vi "Lift_State_Machine.vi"() -> ()   [LabVIEW 2016]
doc: "The state machine for the Lift System.\nDrives the lift forward, then upward, then down, then back to its origin."
uses:
  <vilib>/myRIO/Instrument Drivers/Onboard IO/DIO/typedefs/DIO Reference.ctl
  <vilib>/myRIO/Common/Instrument Driver Framework/Utilities/typedefs/myRIO Generic Hardware Reference.ctl
  <vilib>/myRIO/Common/Instrument Driver Framework/Utilities/typedefs/Hardware Version Enum.ctl
  <vilib>/myRIO/Common/Instrument Driver Framework/Utilities/typedefs/myRIO v1.0 Reference.ctl
  <vilib>/myRIO/Common/Instrument Driver Framework/Utilities/typedefs/Generic FPGA Reference.ctl
  <vilib>/myRIO/Common/Instrument Driver Framework/myRIO v1.0/DIO/typedefs/DIO Channels List.ctl
  <vilib>/myRIO/Common/Instrument Driver Framework/myRIO v1.0/DIO/typedefs/DIO Channels Enum.ctl
  <vilib>/userdefined/High Color/nirio_resource_hc.ctl
  <vilib>/myRIO/Instrument Drivers/Onboard IO/AI/typedefs/AI Reference.ctl
  <vilib>/myRIO/Common/Instrument Driver Framework/myRIO v1.0/AI/typedefs/AI Channels List.ctl
  <vilib>/myRIO/Common/Instrument Driver Framework/myRIO v1.0/AI/typedefs/AI Channels Enum.ctl
  <vilib>/myRIO/Common/Instrument Driver Framework/Utilities/typedefs/Analog Scaling Constants List.ctl
  <vilib>/myRIO/Common/Instrument Driver Framework/Utilities/typedefs/Analog Scaling Constants.ctl
  <vilib>/myRIO/Common/Instrument Driver Framework/Utilities/vis/Is FPGA Ref Available.vi
  <vilib>/myRIO/Common/Instrument Driver Framework/roboRIO v1.0/DIO/vis/roboRIO v1.0 Open DIO.vi
  <vilib>/myRIO/Instrument Drivers/Onboard IO/DIO/vis/Write.vi
  <vilib>/myRIO/Instrument Drivers/Onboard IO/DIO/vis/Read.vi
  <vilib>/myRIO/Common/Instrument Driver Framework/roboRIO v1.0/AI/vis/roboRIO v1.0 Open AI.vi
  <vilib>/myRIO/Instrument Drivers/Onboard IO/AI/vis/Read.vi
  <vilib>/myRIO/Common/Instrument Driver Framework/Utilities/vis/Validate Channels.vi
  <vilib>/myRIO/Common/Instrument Driver Framework/roboRIO v1.0/DIO/vis/roboRIO v1.0 Reserve DIO.vi
  <vilib>/myRIO/Common/Instrument Driver Framework/roboRIO v1.0/AI/vis/roboRIO v1.0 Reserve AI.vi
  <vilib>/myRIO/Common/Instrument Driver Framework/roboRIO v1.0/DIO/vis/roboRIO v1.0 Build MUX Configuration DIO.vi
  <vilib>/myRIO/Common/Instrument Driver Framework/roboRIO v1.0/Resource Manager/vis/roboRIO v1.0 Reserve Channel List.vi
  <vilib>/myRIO/Common/Instrument Driver Framework/roboRIO v1.0/AI/vis/roboRIO v1.0 Build MUX Configuration AI.vi
  <vilib>/myRIO/Common/Instrument Driver Framework/roboRIO v1.0/Resource Manager/vis/roboRIO v1.0 Create Configuration List.vi
  <vilib>/myRIO/Common/Instrument Driver Framework/roboRIO v1.0/Resource Manager/vis/roboRIO v1.0 Reserve Channel.vi
  <vilib>/myRIO/Common/Instrument Driver Framework/roboRIO v1.0/Resource Manager/vis/roboRIO v1.0 Unreserve Channel.vi
  <vilib>/myRIO/Common/Instrument Driver Framework/roboRIO v1.0/Resource Manager/vis/roboRIO v1.0 Build Mutex Name.vi
  <vilib>/Utility/VariantDataType/GetNumericInfo.vi
  <vilib>/Utility/error.llb/Error Cluster From Error Code.vi
  <vilib>/myRIO/Common/Instrument Driver Framework/roboRIO v1.0/roboRIO v1.0 Open.vi
  <vilib>/myRIO/Common/Instrument Driver Framework/Utilities/vis/IO Manager.vi
  <vilib>/myRIO/Common/Instrument Driver Framework/Utilities/vis/Configuration Manager.vi
  <vilib>/myRIO/Common/Instrument Driver Framework/roboRIO v1.0/Resource Manager/vis/roboRIO v1.0 Configure IO.vi
  <vilib>/myRIO/Common/Instrument Driver Framework/myRIO v1.0/myRIO v1.0 Close.vi
  <vilib>/myRIO/Common/Instrument Driver Framework/roboRIO v1.0/DIO/vis/roboRIO v1.0 Write DIO.vi
  <vilib>/myRIO/Common/Instrument Driver Framework/roboRIO v1.0/DIO/vis/roboRIO v1.0 Read DIO.vi
  <vilib>/myRIO/Common/Instrument Driver Framework/roboRIO v1.0/AI/vis/roboRIO v1.0 Get Scaling Constants AI.vi
  <vilib>/myRIO/Common/Instrument Driver Framework/roboRIO v1.0/AI/vis/roboRIO v1.0 Read AI.vi
  <vilib>/myRIO/Express VI/Onboard IO/DO/DO Express VI.xnode
  <vilib>/myRIO/Instrument Drivers/Onboard IO/DIO/vis/myRIO DIO Open.xnode
  <vilib>/myRIO/Express VI/Onboard Devices/Button/Button Express VI.xnode
  <vilib>/myRIO/Express VI/Onboard Devices/LED/LED Express VI.xnode
  <vilib>/myRIO/Express VI/Onboard IO/AI/AI Express VI.xnode
  <vilib>/myRIO/Instrument Drivers/Onboard IO/AI/vis/myRIO AI Open.xnode
  <vilib>/myRIO/Instrument Drivers/Onboard IO/DIO/DIO.lvlib
  <vilib>/myRIO/Instrument Drivers/Onboard IO/AI/AI.lvlib
panel:
  in  "State change delay":dbl=1.0 caption="Delay Time (s)"
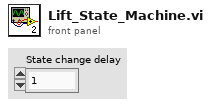
[diagram p1: front panel]
types:
  T1 = typedef "DIO.lvlib/DIO Reference.ctl" = cluster{"myRIO Reference":T2, "DIO Channels List":T6}
  T2 = typedef "myRIO Generic Hardware Reference.ctl" = cluster{"myRIO Model":T3, "myRIO Hardware Reference":T4}
  T3 = typedef "Hardware Version Enum.ctl" = enum16{"Unknown", "myRIO-1900", "myRIO-1950", "roboRIO", "NI ELVIS RIO CM"}
  T4 = typedef "myRIO v1.0 Reference.ctl" = cluster{"Generic FPGA Reference":T5, "Allow multiple opens":bool}
  T5 = typedef "Generic FPGA Reference.ctl" = refnum<k20>
  T6 = typedef "DIO Channels List.ctl" = T7[]
  T7 = typedef "DIO Channels Enum.ctl" = enum16{"Not Connected", "C/DIO0", "C/DIO1", "C/DIO2", "C/DIO3", "C/DIO4", "C/DIO5", "C/DIO6", "C/DIO7", "A/DIO0", "A/DIO1", "A/DIO2", "A/DIO3", "A/DIO4", "A/DIO5", "A/DIO6", "A/DIO7", "A/DIO8", "A/DIO9", "A/DIO10", "A/DIO11", "A/DIO12", "A/DIO13", "A/DIO14", "A/DIO15", "B/DIO0", "B/DIO1", "B/DIO2", "B/DIO3", "B/DIO4", "B/DIO5", "B/DIO6", "B/DIO7", "B/DIO8", "B/DIO9", "B/DIO10", "B/DIO11", "B/DIO12", "B/DIO13", "B/DIO14", "B/DIO15", "LED0", "LED1", "LED2", "LED3", "Button0", "DIO/DIO0", "DIO/DIO1", "DIO/DIO2", "DIO/DIO3", "DIO/DIO4", "DIO/DIO5", "DIO/DIO6", "DIO/DIO7", "DIO/DIO8", "DIO/DIO9", "SPI/CS0", "SPI/CS1", "SPI/CS2", "SPI/CS3", "LED RADIO (Green)", "LED RADIO (Red)", "LED COMM (Green)", "LED COMM (Red)", "LED MODE (Green)", "LED MODE (Red)"}
  T8 = typedef "nirio_resource_hc.ctl" = tag
  T9 = typedef "AI.lvlib/AI Reference.ctl" = cluster{"myRIO Reference":T2, "AI Channels List":T10, "AI Scaling Constants List":T12}
  T10 = typedef "AI Channels List.ctl" = T11[]
  T11 = typedef "AI Channels Enum.ctl" = enum16{"Not Connected", "AudioIn/Left", "AudioIn/Right", "C/AI0", "C/AI1", "A/AI0", "A/AI1", "A/AI2", "A/AI3", "B/AI0", "B/AI1", "B/AI2", "B/AI3", "AI/AI0", "AI/AI1", "AI/AI2", "AI/AI3"}
  T12 = typedef "Analog Scaling Constants List.ctl" = T13[]
  T13 = typedef "Analog Scaling Constants.ctl" = cluster{"LSB Weight (Volts)":dbl, "Offset (Volts)":dbl, "Signed?":bool}
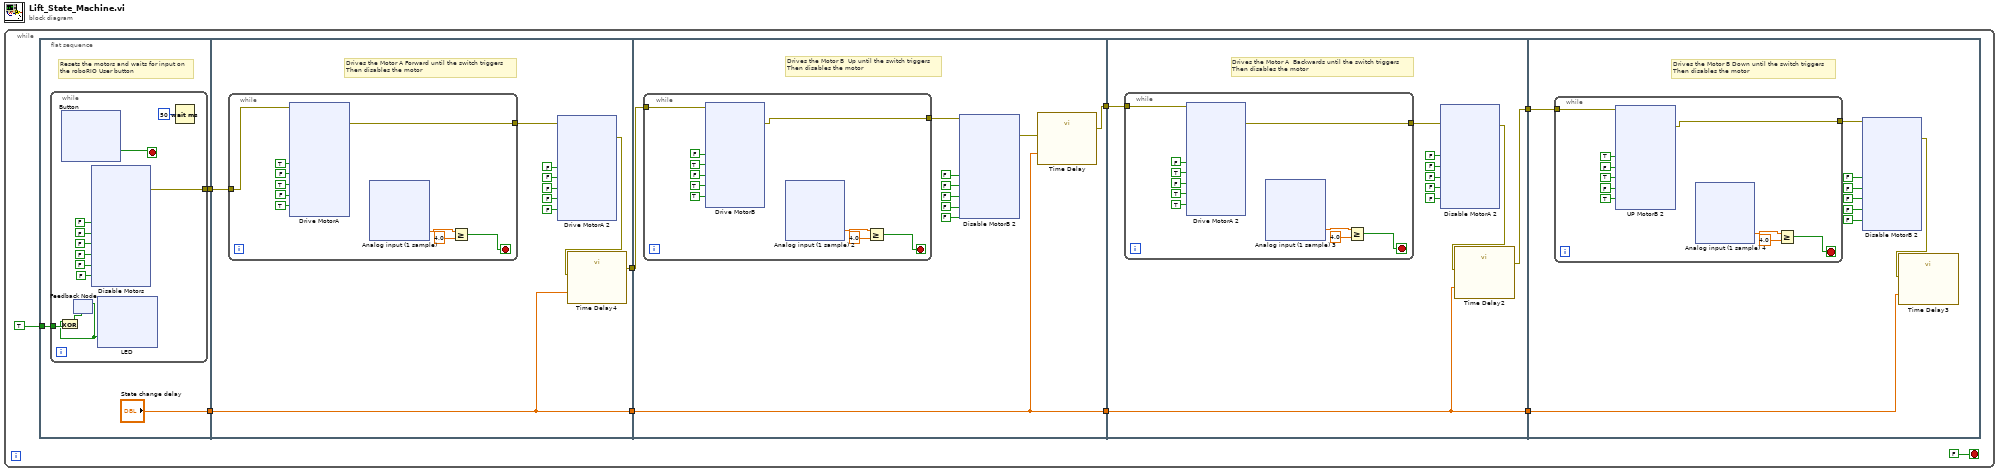
[diagram p0: block diagram]
diagram:
  n1 = while {
    stop <- FALSE stop-if-true
    n2 = flat-sequence {
      tunnel: ["State change delay"] -> w10
      tunnel: [w12] -> w9
      tunnel: TRUE -> [w11]
      tunnel: w10 -> [w138]
      tunnel: [w138] -> w8
      tunnel: [w137] -> w7
      tunnel: w9 -> [w136]
      tunnel: w8 -> [w273]
      tunnel: [w273] -> w6
      tunnel: w7 -> [w272]
      tunnel: [w271] -> w5
      tunnel: w6 -> [w408]
      tunnel: [w408] -> w4
      tunnel: w5 -> [w407]
      tunnel: [w406] -> w3
      tunnel: w4 -> [w542]
      tunnel: w3 -> [w541]
      frame #0 {
        # "Resets the motors and waits for input on\nthe roboRIO User button"
        n3 = while {
          tunnel: [w19] -> w12
          tunnel: w11 -> [w17]
          stop <- w18 stop-if-true
          n4 = xnode "Button"() -> ("Value"=w18:bool)  [unwired: 1 in, 1 out]
          n5 = feedback #1() -> (w15:bool)  [unwired: 1 in]
          n6 = Exclusive Or(1:w17, 2:w15) -> (0:w16:bool)
          n7 = feedback-in #1(w16) -> ()
          n8 = xnode "Disable Motors"("IN1 (B/DIO0 (Pin 11))"=FALSE, "IN2 (B/DIO1 (Pin 13))"=FALSE, "IN3 (B/DIO2 (Pin 15))"=FALSE, "IN4 (B/DIO3 (Pin 17))"=FALSE, "ENABLE A (B/DIO13 (Pin 26))"=FALSE, "ENABLE B (B/DIO8 (Pin 27))"=FALSE) -> ("error out"=w19:errorcluster)  [unwired: 1 in]
          n9 = xnode "LED"("COMM (Green)"=w15) -> ()  [unwired: 1 in, 1 out]
          n10 = Wait (ms)(milliseconds to wait=u32 50) -> ()  [unwired: 1 out]
        }
      }
      frame #1 {
        # "Drives the Motor A Forward until the switch triggers\nThen disables the motor"
        n11 = while {
          tunnel: [w187] -> w140
          tunnel: w136 -> [w185]
          stop <- w188 stop-if-true
          n12 = xnode "Drive MotorA"("IN1 (B/DIO0 (Pin 11))"=TRUE, "IN2 (B/DIO1 (Pin 13))"=FALSE, "IN3 (B/DIO2 (Pin 15))"=TRUE, "IN4 (B/DIO3 (Pin 17))"=FALSE, "ENABLE A (B/DIO13 (Pin 26))"=TRUE, "error in (no error)"=w185) -> ("error out"=w187:errorcluster)
          n13 = xnode "Analog input (1 sample)"() -> ("B/AI1 (Pin 5)"=w186:dbl)  [unwired: 1 in, 1 out]
          n14 = Greater Or Equal?(x=w186, y=4.0) -> (x >= y?=w188:bool)
        }
        n15 = xnode "Drive MotorA 2"("IN1 (B/DIO0 (Pin 11))"=FALSE, "IN2 (B/DIO1 (Pin 13))"=FALSE, "IN3 (B/DIO2 (Pin 15))"=FALSE, "IN4 (B/DIO3 (Pin 17))"=FALSE, "ENABLE A (B/DIO13 (Pin 26))"=FALSE, "error in (no error)"=w140) -> ("error out"=w139:errorcluster)
        n16 = call "Time Delay4"("error in (no error)"=w139, "Delay Time (s)"=w138) -> ("error out"=w137:errorcluster)  [unwired: 9 in]
      }
      frame #2 {
        # "Drives the Motor B  Up until the switch triggers\nThen disables the motor"
        n17 = while {
          tunnel: [w322] -> w275
          tunnel: w272 -> [w320]
          stop <- w324 stop-if-true
          n18 = xnode "Drive MotorB"("IN1 (B/DIO0 (Pin 11))"=FALSE, "IN2 (B/DIO1 (Pin 13))"=TRUE, "IN3 (B/DIO2 (Pin 15))"=FALSE, "IN4 (B/DIO3 (Pin 17))"=TRUE, "ENABLE B (B/DIO8 (Pin 27))"=TRUE ("ENABLE A (B/DIO13 (Pin 26))"), "error in (no error)"=w320) -> ("error out"=w322:errorcluster)
          n19 = xnode "Analog input (1 sample) 2"() -> ("B/AI3 (Pin 9)"=w321:dbl)  [unwired: 1 in, 1 out]
          n20 = Greater Or Equal?(x=w321, y=4.0) -> (x >= y?=w324:bool)
        }
        n21 = xnode "Disable MotorB 2"("IN1 (B/DIO0 (Pin 11))"=FALSE, "IN2 (B/DIO1 (Pin 13))"=FALSE, "IN3 (B/DIO2 (Pin 15))"=FALSE, "IN4 (B/DIO3 (Pin 17))"=FALSE, "ENABLE B (B/DIO8 (Pin 27))"=FALSE ("ENABLE A (B/DIO13 (Pin 26))"), "error in (no error)"=w275) -> ("error out"=w274:errorcluster)
        n22 = call "Time Delay"("error in (no error)"=w274, "Delay Time (s)"=w273) -> ("error out"=w271:errorcluster)  [unwired: 9 in]
      }
      frame #3 {
        # "Drives the Motor A  Backwards until the switch triggers\nThen disables the motor"
        n23 = while {
          tunnel: [w457] -> w410
          tunnel: w407 -> [w455]
          stop <- w458 stop-if-true
          n24 = xnode "Drive MotorA 2"("IN1 (B/DIO0 (Pin 11))"=FALSE, "IN2 (B/DIO1 (Pin 13))"=TRUE, "IN3 (B/DIO2 (Pin 15))"=FALSE, "IN4 (B/DIO3 (Pin 17))"=TRUE, "ENABLE A (B/DIO13 (Pin 26))"=TRUE, "error in (no error)"=w455) -> ("error out"=w457:errorcluster)
          n25 = xnode "Analog input (1 sample) 3"() -> ("B/AI0 (Pin 3)"=w456:dbl)  [unwired: 1 in, 1 out]
          n26 = Greater Or Equal?(x=w456, y=4.0) -> (x >= y?=w458:bool)
        }
        n27 = xnode "Disable MotorA 2"("IN1 (B/DIO0 (Pin 11))"=FALSE, "IN2 (B/DIO1 (Pin 13))"=FALSE, "IN3 (B/DIO2 (Pin 15))"=FALSE, "IN4 (B/DIO3 (Pin 17))"=FALSE, "ENABLE A (B/DIO13 (Pin 26))"=FALSE, "error in (no error)"=w410) -> ("error out"=w409:errorcluster)
        n28 = call "Time Delay2"("error in (no error)"=w409, "Delay Time (s)"=w408) -> ("error out"=w406:errorcluster)  [unwired: 9 in]
      }
      frame #4 {
        # "Drives the Motor B Down until the switch triggers\nThen disables the motor"
        n29 = while {
          tunnel: [w591] -> w544
          tunnel: w541 -> [w589]
          stop <- w593 stop-if-true
          n30 = xnode "UP MotorB 2"("IN1 (B/DIO0 (Pin 11))"=TRUE, "IN2 (B/DIO1 (Pin 13))"=FALSE, "IN3 (B/DIO2 (Pin 15))"=TRUE, "IN4 (B/DIO3 (Pin 17))"=FALSE, "ENABLE B (B/DIO8 (Pin 27))"=TRUE ("ENABLE A (B/DIO13 (Pin 26))"), "error in (no error)"=w589) -> ("error out"=w591:errorcluster)
          n31 = xnode "Analog input (1 sample) 4"() -> ("B/AI2 (Pin 7)"=w590:dbl)  [unwired: 1 in, 1 out]
          n32 = Greater Or Equal?(x=w590, y=4.0) -> (x >= y?=w593:bool)
        }
        n33 = xnode "Disable MotorB 2"("IN1 (B/DIO0 (Pin 11))"=FALSE, "IN2 (B/DIO1 (Pin 13))"=FALSE, "IN3 (B/DIO2 (Pin 15))"=FALSE, "IN4 (B/DIO3 (Pin 17))"=FALSE, "ENABLE B (B/DIO8 (Pin 27))"=FALSE ("ENABLE A (B/DIO13 (Pin 26))"), "error in (no error)"=w544) -> ("error out"=w543:errorcluster)
        n34 = call "Time Delay3"("error in (no error)"=w543, "Delay Time (s)"=w542) -> ()  [unwired: 9 in, 1 out]
      }
    }
  }
